vi "DelayDiscounting.vi"() -> ()   [LabVIEW 2009]
uses:
  <vilib>/Utility/file.llb/Write To Spreadsheet File (string).vi
panel:
  out "interface\nstate":enum32{"prompt", "trials"}(tab)
  in  "OK Button":bool
  out "information":string="hello."
  out "trial text":string
  in  "Left":bool
  in  "Right":bool
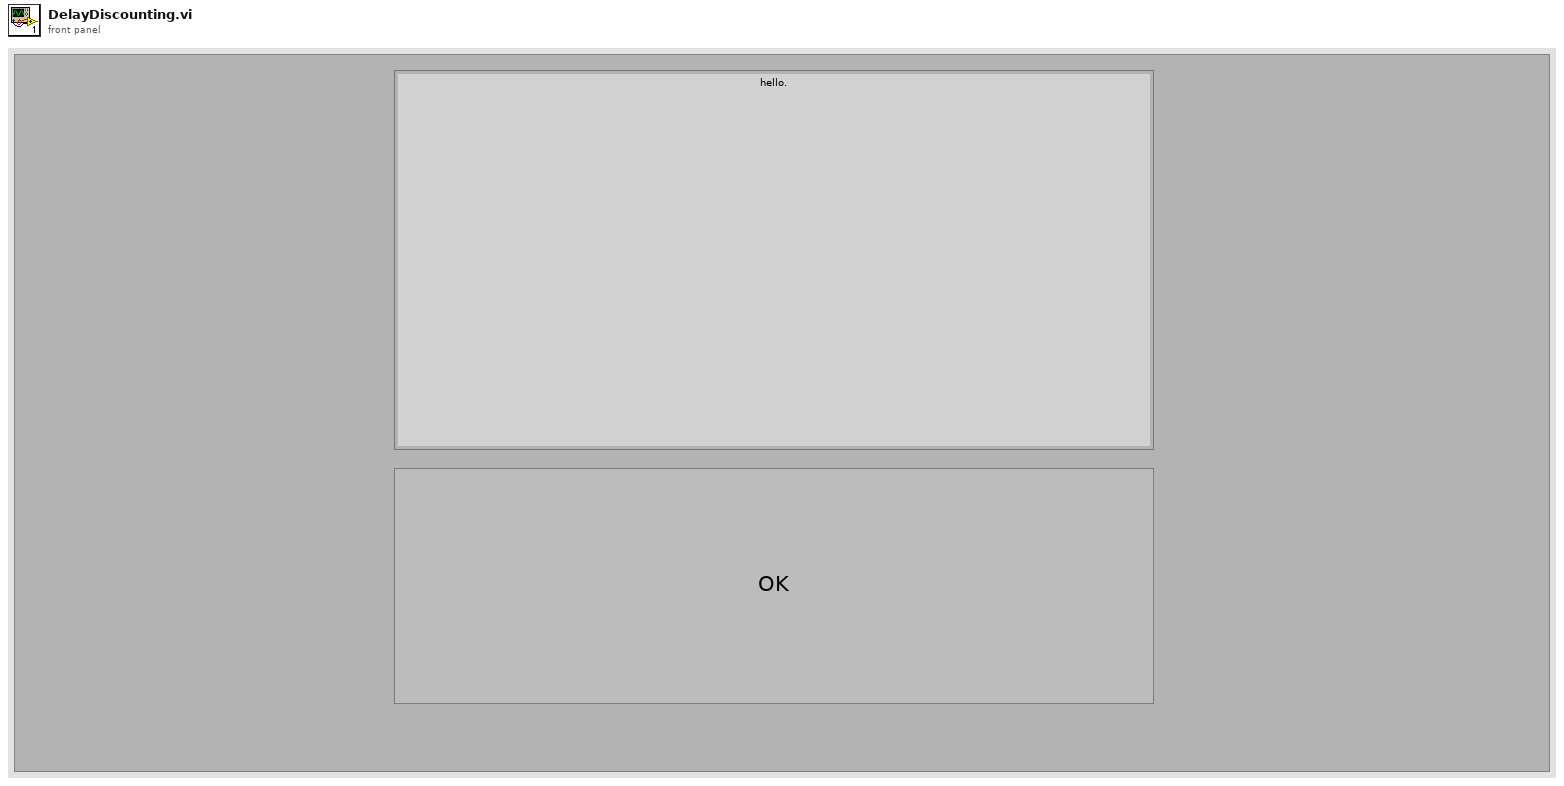
[diagram p1: front panel]
types:
  T1 = cluster{"interface type":enum16{"prompt", "trials"}, "section description":string, "text":string, "LLR delays":string[], "LLR prefix":string, "LLR unit":string, "LLR magnitude":i32, "titrations":i32}[]
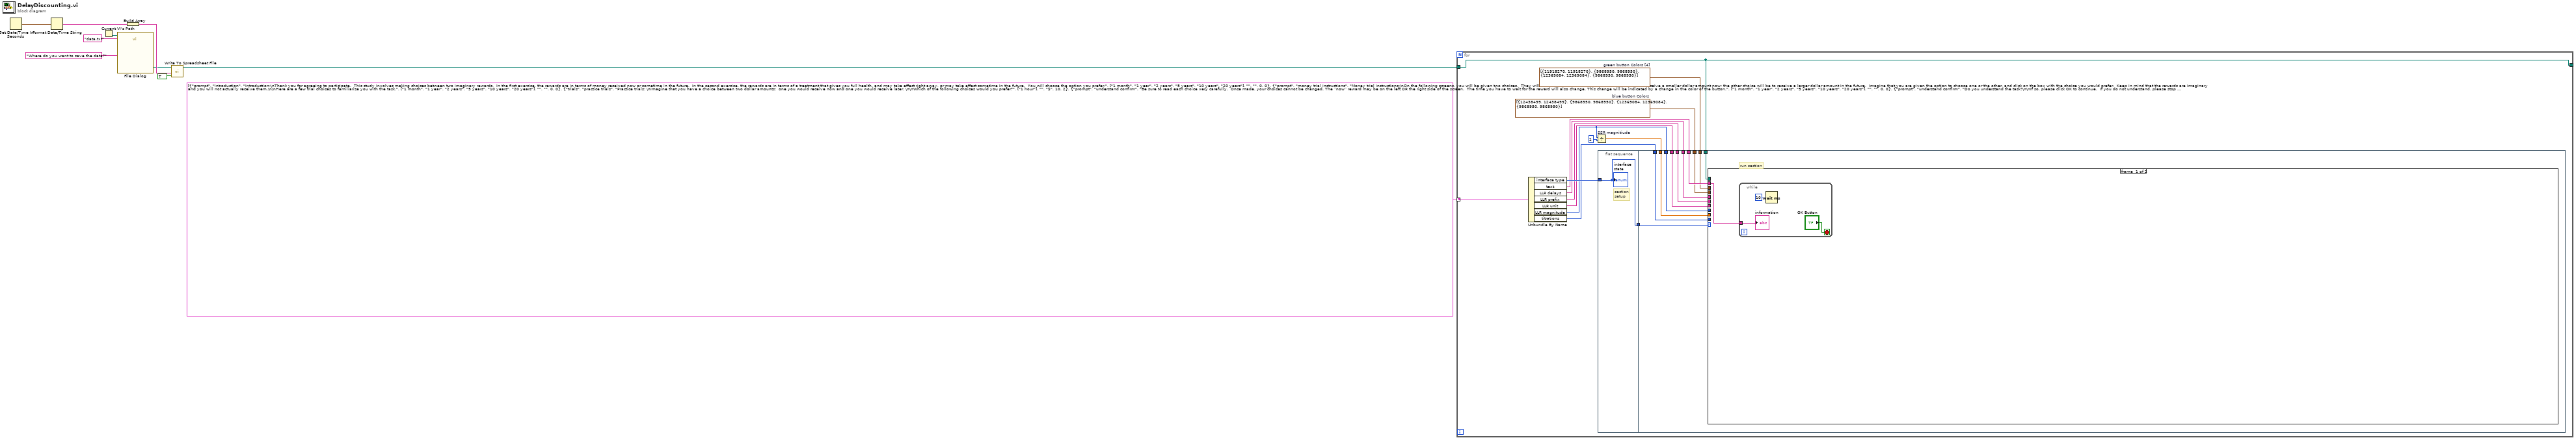
[diagram p0: block diagram]
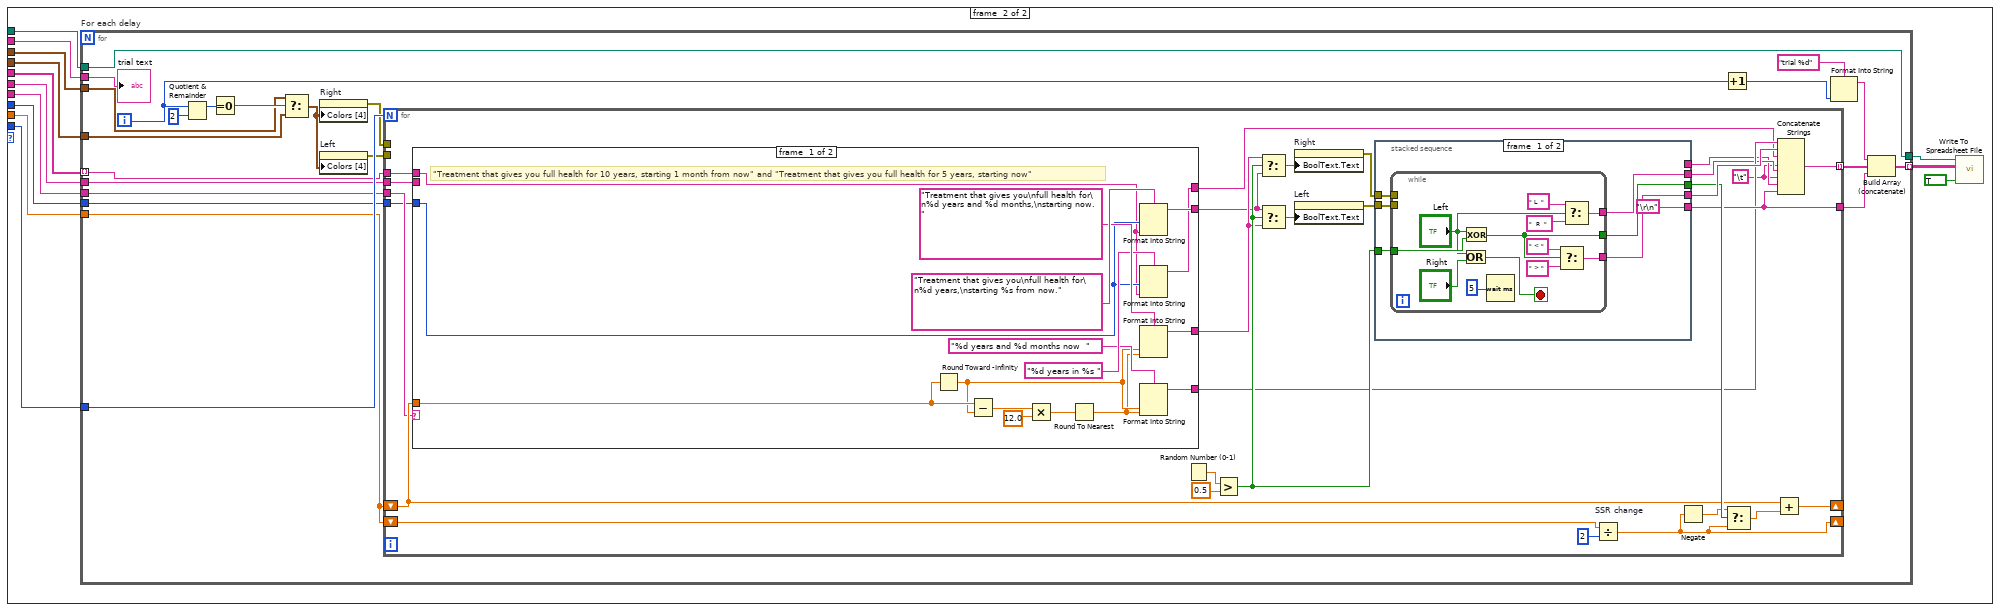
[diagram p2: hidden frame]
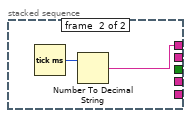
[diagram p3: hidden frame]
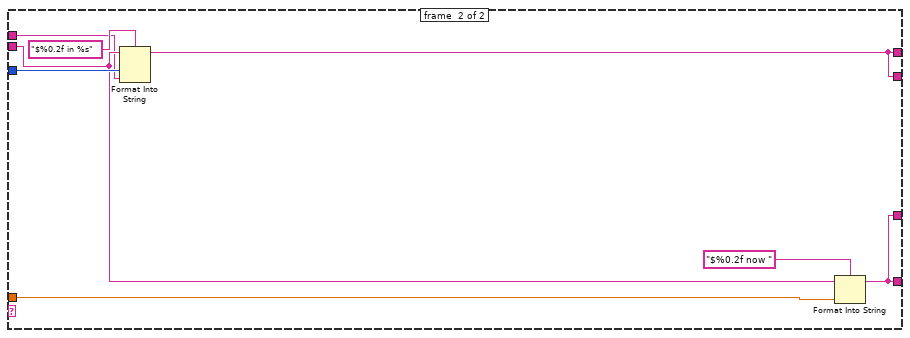
[diagram p4: hidden frame]
diagram:
  n1 = Get Date/Time In Seconds() -> (seconds since 1Jan1904=w6:timestamp)
  n2 = Format Date/Time String(seconds (now)=w6) -> (date/time string=w5:string)  [unwired: 2 in]
  n3 = Current VI's Path() -> (path=w7:path)
  n4 = call "File Dialog"("start path"=w7, "prompt"="Where do you want to save the data?", "default name"="data.txt") -> ("selected path"=w2:path)  [unwired: 9 in, 3 out]
  n5 = Build Array(w5) -> (w4:string[])
  n6 = call-poly <vilib>:"Write To Spreadsheet File.vi"("append to file? (new file:F)"=TRUE, "1D data"=w4, "file path (dialog if empty)"=w2) -> ("new file path (Not A Path if cancelled)"=w1:path)  [unwired: 5 in]
  n7 = for {
    tunnel: T1 [{"interface type"=enum."prompt", "section description"="introduction", "text"="Introduction:\nThank you for agreeing to participate.  This study involves making choices between two imaginary rewards.  In the first exercise, the rewards are in terms of money received now or sometime in the future.  In the second exercise, the rewards are in terms of a treatment that gives you full health, and may take effect right away, or may take effect sometime in the future.  You will choose the option you prefer.", "LLR delays"=["1 month", "1 year", "2 years", "5 years", "10 years", "20 years"], "LLR prefix"="", "LLR unit"="", "LLR magnitude"=0, "titrations"=0}, {"interface type"=enum."prompt", "section description"="money trial instructions", "text"="Money trial instructions:\nOn the following screens, you will be given two choices.  They will have different dollar values.  One choice will be to receive a smaller dollar amount now; the other choice will be to receive a larger dollar amount in the future.  Imagine that you are given the option to choose one or the other, and click on the box with the choice you would prefer.  Keep in mind that the rewards are imaginary and you will not actually receive them.\n\nHere are a few trial choices to familiarize you with the task.", "LLR delays"=["1 month", "1 year", "2 years", "5 years", "10 years", "20 years"], "LLR prefix"="", "LLR unit"="", "LLR magnitude"=0, "titrations"=0}, {"interface type"=enum."trials", "section description"="practice trials", "text"="Practice trials: \nImagine that you have a choice between two dollar amounts:  one you would receive now and one you would receive later. \n\nWhich of the following choices would you prefer?", "LLR delays"=["1 hour"], "LLR prefix"="", "LLR unit"="$", "LLR magnitude"=10, "titrations"=2}, {"interface type"=enum."prompt", "section description"="understand confirm", "text"="Be sure to read each choice very carefully.  Once made, your choices cannot be changed. The “now” reward may be on the left OR the right side of the screen.  The time you have to wait for the reward will also change. This change will be indicated by a change in the color of the button.", "LLR delays"=["1 month", "1 year", "2 years", "5 years", "10 years", "20 years"], "LLR prefix"="", "LLR unit"="", "LLR magnitude"=0, "titrations"=0}, {"interface type"=enum."prompt", "section description"="understand confirm", "text"="Do you understand the task?\n\nIf so, please click OK to continue.  If you do not understand, please stop now and ask the researcher for further assistance.", "LLR delays"=["1 month", "1 year", "2 years", "5 years", "10 years", "20 years"], "LLR prefix"="", "LLR unit"="", "LLR magnitude"=0, "titrations"=0}, {"interface type"=enum."prompt", "section description"="understand confirm", "text"="Remember:\nYou cannot go back. You cannot change your choices after you make them.", "LLR delays"=["1 month", "1 year", "2 years", "5 years", "10 years", "20 years"], "LLR prefix"="", "LLR unit"="", "LLR magnitude"=0, "titrations"=0}, {"interface type"=enum."trials", "section description"="money trials", "text"="Imagine that you have a choice between two dollar amounts:  one you would receive now and one you would receive later. \n\nWhich of the following choices would you prefer?", "LLR delays"=["1 month", "1 year", "2 years", "5 years", "10 years", "20 years"], "LLR prefix"="", "LLR unit"="$", "LLR magnitude"=1000, "titrations"=6}, {"interface type"=enum."prompt", "section description"="health trial instructions", "text"="Health trial instructions:\nOn the next screen, you will see a health scenario.  Read the scenario and imagine yourself in that condition.\n\nOn the following screens, you will be given two choices of treatments for this imaginary health condition.\n\nBoth treatments return you to full health.  One treatment will return you to full health starting now.  The other treatment will return you to full health for a longer period of time – but will not take effect until sometime in the future.\n\nClick on the box with the choice you would prefer.", "LLR delays"=["1 week"], "LLR prefix"="", "LLR unit"="", "LLR magnitude"=0, "titrations"=6}, {"interface type"=enum."prompt", "section description"="health trials senario", "text"="Imagine that for the past two years your state of health has fit this description:\n\nBecause of your doctor’s instructions, you need to take multiple medications each day.  To monitor the effects of these medications, you must get blood drawn at your doctor’s office at least once per month.  You must also be very careful about what you eat and drink.  You have to limit the amount of salt you eat and fluids you drink.  You often have swollen ankles.  You sometimes have chest pain, for which you must take nitroglycerin tablets.  You have to visit the bathroom often to urinate.  You often feel tired and cannot walk more than 20 feet without getting short of breath.  You often do not have the energy for sexual activity.  Sometimes, you feel depressed about your health.\n", "LLR delays"=["1 month", "1 year", "2 years", "5 years", "10 years", "20 years"], "LLR prefix"="", "LLR unit"="", "LLR magnitude"=0, "titrations"=0}, {"interface type"=enum."trials", "section description"="practice trials", "text"="Practice trials:\n\nImagine that you have a choice between two treatments which return you to full health for different amounts of time and will take effect starting now or at some point in the future.\n\nWhich of the following choices would you prefer?", "LLR delays"=["1 hour"], "LLR prefix"="", "LLR unit"="years", "LLR magnitude"=10, "titrations"=2}, {"interface type"=enum."prompt", "section description"="understand confirm", "text"="Be sure to read each choice very carefully.  The “now” treatment may be on the left OR the right side of the screen.  The time you have to wait for the treatment to take effect will also change.\n\nYou cannot change your choice after it has been clicked.", "LLR delays"=["1 month", "1 year", "2 years", "5 years", "10 years", "20 years"], "LLR prefix"="", "LLR unit"="", "LLR magnitude"=0, "titrations"=0}, {"interface type"=enum."prompt", "section description"="understand confirm", "text"="Do you understand the task?\n\nIf so, please click OK to continue.  If you do not understand, please stop now and ask the researcher for further assistance.", "LLR delays"=["1 month", "1 year", "2 years", "5 years", "10 years", "20 years"], "LLR prefix"="", "LLR unit"="", "LLR magnitude"=0, "titrations"=0}, {"interface type"=enum."trials", "section description"="health trials", "text"="Imagine that you have a choice between two treatments which return you to full health for different amounts of time and will take effect starting now or at some point in the future.\n\nWhich of the following choices would you prefer?", "LLR delays"=["1 month", "1 year", "2 years", "5 years", "10 years", "20 years"], "LLR prefix"="", "LLR unit"="years", "LLR magnitude"=10, "titrations"=6}, {"interface type"=enum."prompt", "section description"="the end", "text"="Thank you, the experiment is done. Please inform the researcher.", "LLR delays"=["1 month", "1 year", "2 years", "5 years", "10 years", "20 years"], "LLR prefix"="", "LLR unit"="", "LLR magnitude"=0, "titrations"=0}] -> [w24] mode=indexing
    tunnel: w1 -> [w17]
    tunnel: [w17] -> _
    w11 = cluster{u32, u32}[] [{11918270, 11918270}, {9868950, 9868950}, {12369084, 12369084}, {9868950, 9868950}]  # green button Colors [4]
    w12 = cluster{u32, u32}[] [{12438499, 12438499}, {9868950, 9868950}, {12369084, 12369084}, {9868950, 9868950}]  # blue button Colors
    n8 = Unbundle By Name(w24) -> ("interface type"=w23:enum16{"prompt", "trials"}, "text"=w21:string, "LLR delays"=w19:string[], "LLR prefix"=w14:string, "LLR unit"=w13:string, "LLR magnitude"=w15:i32, "titrations"=w18:i32)
    n9 = Divide "SSR magnitiude"(x=w15, y=2) -> (x/y=w16:dbl)
    n10 = flat-sequence {
      tunnel: w23 -> [w25]
      tunnel: [w25] -> w22
      tunnel: w22 -> [w36]
      tunnel: w21 -> [w35]
      tunnel: w19 -> [w34]
      tunnel: w18 -> [w33]
      tunnel: w17 -> [w32]
      tunnel: w16 -> [w31]
      tunnel: w15 -> [w30]
      tunnel: w14 -> [w29]
      tunnel: w13 -> [w28]
      tunnel: w12 -> [w27]
      tunnel: w11 -> [w26]
      frame #0 {
        # "section\nsetup"
        "interface\nstate" <- w25
      }
      frame #1 {
        # "run section"
        n11 = case shown="\"trials\"" w36 {
          tunnel: w35 -> [w37 w53]
          tunnel: w34 -> [_ w52]
          tunnel: w33 -> [_ w51]
          tunnel: w32 -> [_ w50]
          tunnel: w31 -> [_ w49]
          tunnel: w30 -> [_ w48]
          tunnel: w29 -> [_ w47]
          tunnel: w28 -> [_ w43]
          tunnel: w27 -> [_ w41]
          tunnel: w26 -> [_ w42]
          frame #0 {
            n12 = while {
              tunnel: w37 -> [w39]
              stop <- "OK Button" stop-if-true
              n13 = Wait (ms)(milliseconds to wait=u32 10) -> ()  [unwired: 1 out]
              "information" <- w39
            }
          }
          frame #1 {
            n14 = for "For each delay" {
              tunnel: w53 -> [w76]
              tunnel: w52 -> [w63] mode=indexing
              tunnel: w51 -> [w75]
              tunnel: w50 -> [w71]
              tunnel: w49 -> [w64]
              tunnel: w48 -> [w74]
              tunnel: w47 -> [w73]
              tunnel: w43 -> [w72]
              tunnel: [w70] -> w46 mode=indexing
              tunnel: [w71] -> w45
              tunnel: w42 -> [w57]
              tunnel: w41 -> [w56]
              i -> [w58]
              n15 = Quotient & Remainder(x=w58, y=2) -> (x-y*floor(x/y)=w60:i32)  [unwired: 1 out]
              n16 = Equal To 0?(x=w60) -> (x = 0?=w62:bool)
              n17 = Select(t=w57, s=w62, f=w56) -> (s? t:f=w59:cluster{u32, u32}[])
              n18 = property on="Right" class="Bool"("Colors [4]"=w59) -> (error out=w55:errorcluster)  [unwired: 2 in, 1 out]
              n19 = property on="Left" class="Bool"("Colors [4]"=w59) -> (error out=w54:errorcluster)  [unwired: 2 in, 1 out]
              n20 = for {
                N: w75 -> [_]
                tunnel: [w102] -> w67 mode=indexing
                tunnel: w74 -> [w84]
                tunnel: w73 -> [w101]
                tunnel: w72 -> [w85]
                shift-right: [w97] -> _
                shift-left: w64 -> [w93]
                tunnel: [w95] -> w66
                shift-right: [w94] -> _
                shift-left: w64 -> [w92]
                tunnel: w63 -> [w83]
                tunnel: w55 -> [_]
                tunnel: w54 -> [_]
                w77 = "\t"
                n21 = case shown="\"years\"" w85 {
                  tunnel: w101 -> [_ w146]
                  tunnel: w93 -> [w137 w149]
                  tunnel: [w136 w144] -> w86
                  tunnel: w84 -> [w133 w147]
                  tunnel: w83 -> [w132 w145]
                  tunnel: [w135 w143] -> w82
                  tunnel: [w127 w144] -> w81
                  tunnel: [w131 w143] -> w80
                  frame #0 {
                    # "\"Treatment that gives you full health for 10 years, starting 1 month from now\" and \"Treatment that gives you full health for 5 years, starting now\""
                    n22 = Round Toward -Infinity(1:w137) -> (0:w129:dbl)
                    n23 = Subtract(x=w137, y=w129) -> (x-y=w142:dbl)
                    n24 = Multiply(x=w142, y=12.0) -> (x*y=w140:dbl)
                    n25 = Round To Nearest(number=w140) -> (nearest integer value=w128:dbl)
                    n26 = Format Into String(format string="Treatment that gives you\nfull health for\n%d years,\nstarting %s from now.", w133, w132) -> (resulting string=w135:string)  [unwired: 2 in, 1 out]
                    n27 = Format Into String(format string="%d years in %s ", w133, w132) -> (resulting string=w131:string)  [unwired: 2 in, 1 out]
                    n28 = Format Into String(format string="Treatment that gives you\nfull health for\n%d years and %d months,\nstarting now.", w129, w128) -> (resulting string=w136:string)  [unwired: 2 in, 1 out]
                    n29 = Format Into String(format string="%d years and %d months now  ", w129, w128) -> (resulting string=w127:string)  [unwired: 2 in, 1 out]
                  }
                  frame #1 {
                    n30 = Format Into String(format string="$%0.2f in %s", initial string=w146, w147, w145) -> (resulting string=w143:string)  [unwired: 1 in, 1 out]
                    n31 = Format Into String(format string="$%0.2f now ", initial string=w146, w149) -> (resulting string=w144:string)  [unwired: 1 in, 1 out]
                  }
                }
                n32 = Random Number (0-1)() -> (number: 0 to 1=w91:dbl)
                n33 = Greater?(x=w91, y=0.5) -> (0:w87:bool)
                n34 = Select(t=w86, s=w87, f=w82) -> (s? t:f=w88:string)
                n35 = Select(t=w82, s=w87, f=w86) -> (s? t:f=w89:string)
                n36 = property on="Right" class="Bool"("BoolText.Text"=w88) -> (error out=w104:errorcluster)  [unwired: 2 in, 1 out]
                n37 = property on="Left" class="Bool"("BoolText.Text"=w89) -> (error out=w105:errorcluster)  [unwired: 2 in, 1 out]
                n38 = stacked-sequence {
                  tunnel: w105 -> [w112 _]
                  tunnel: w104 -> [w111 _]
                  tunnel: [w110 _] -> w103
                  tunnel: [w109 _] -> w99
                  tunnel: ["\r\n" _] -> w95
                  tunnel: w87 -> [w107 _]
                  tunnel: [w106 _] -> w79
                  tunnel: [_ w125] -> w78
                  frame #0 {
                    n39 = while {
                      tunnel: w112 -> [_]
                      tunnel: w111 -> [_]
                      tunnel: [w119] -> w110
                      tunnel: [w118] -> w109
                      tunnel: w107 -> [w117]
                      tunnel: [w114] -> w106
                      stop <- w122 stop-if-true
                      n40 = Or(x="Left", y="Right") -> (x .or. y?=w122:bool)
                      n41 = Exclusive Or(1:w117, 2:"Left") -> (0:w118:bool)
                      n42 = Wait (ms)(milliseconds to wait=u32 5) -> ()  [unwired: 1 out]
                      n43 = Select(t=" < ", s=w118, f=" > ") -> (s? t:f=w119:string)
                      n44 = Select(t=" L  ", s="Left", f="  R  ") -> (s? t:f=w114:string)
                    }
                  }
                  frame #1 {
                    n45 = Tick Count (ms)() -> (millisecond timer value=w126:u32)
                    n46 = Number To Decimal String(number=w126) -> (decimal integer string=w125:string)  [unwired: 1 in]
                  }
                }
                n47 = Divide "SSR change"(x=w92, y=2) -> (x/y=w94:dbl)
                n48 = Negate(x=w94) -> (-x=w96:dbl)
                n49 = Select(t=w96, s=w99, f=w94) -> (s? t:f=w98:dbl)
                n50 = Add(x=w93, y=w98) -> (x+y=w97:dbl)
                n51 = Concatenate Strings(w81, w103, w80, w77, w79, w77, w78, w95) -> (w102:string)
              }
              n52 = Increment(x=w58) -> (x+1=w65:i32)
              n53 = Format Into String(format string="trial %d", w65) -> (resulting string=w68:string)  [unwired: 2 in, 1 out]
              n54 = Build Array (concatenate)(w68, w67, w66) -> (w70:string[])
              "trial text" <- w76
            }
            n55 = call-poly <vilib>:"Write To Spreadsheet File.vi"("append to file? (new file:F)"=TRUE, "2D data"=w46, "file path (dialog if empty)"=w45) -> ()  [unwired: 5 in, 1 out]
          }
        }
      }
    }
  }
